vi "control_excitadores.vi"(4 "Action":u32, 5 "AL TX 1":bool caption="AL TX", 7 "COM DATA":T1={"IP "="192.168.1.7", "Puerto:"=2101, "Time Out"=800}) -> (1 "error out":errorcluster)   [LabVIEW 2010]
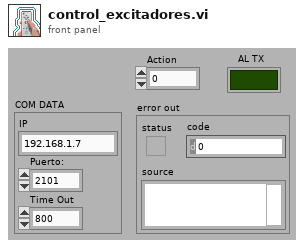
[diagram p1: front panel]
types:
  T1 = cluster{"IP ":string, "Puerto:":u16, "Time Out":u16}
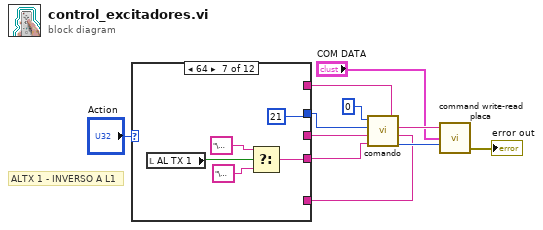
[diagram p0: block diagram]
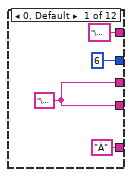
[diagram p2: hidden frame]
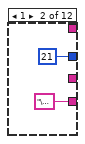
[diagram p3: hidden frame]
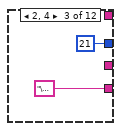
[diagram p4: hidden frame]
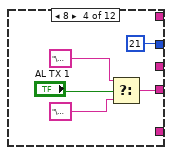
[diagram p5: hidden frame]
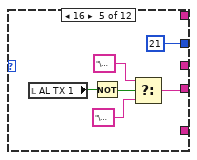
[diagram p6: hidden frame]
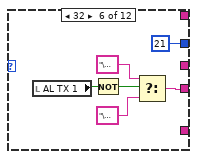
[diagram p7: hidden frame]
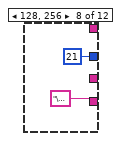
[diagram p8: hidden frame]
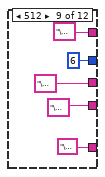
[diagram p9: hidden frame]
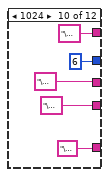
[diagram p10: hidden frame]
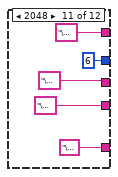
[diagram p11: hidden frame]
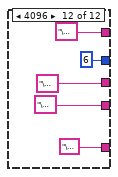
[diagram p12: hidden frame]
diagram:
  # "ALTX 1 - INVERSO A L1"
  n1 = case shown="64" "Action" {
    tunnel: [w15 _ _ _ _ _ _ _ "\u0003" ("ANEXO H") "\u0003" ("ANEXO H") "\u0003" ("ANEXO H") "\u0003" ("ANEXO H")] -> w6
    tunnel: [w15 "\u0006" ("LOW") "\u0007" ("LOW") w20 w26 w31 w37 "\u0001" ("LOW") "\u0000" ("ANEXO H") "\u0000" ("ANEXO H") "\u0000" ("ANEXO H") "\u0000" ("ANEXO H")] -> w5
    tunnel: ["\u0004" ("ANEXO H") _ _ _ _ _ _ _ "\u0000" ("ANEXO H") "\u0001" ("ANEXO H") "\u0002" ("ANEXO H") "\u0003" ("ANEXO H")] -> w4
    tunnel: ["À" ("LOW") _ _ _ _ _ _ _ "\u0000" ("LOW") "\u0000" ("LOW") "\u0000" ("LOW") "\u0000" ("LOW")] -> w3
    tunnel: [u8 6 ("Comando:") u8 21 ("Comando:") u8 21 ("Comando:") u8 21 ("Comando:") u8 21 ("Comando:") u8 21 ("Comando:") u8 21 ("Comando:") u8 21 ("Comando:") u8 6 ("Comando:") u8 6 ("Comando:") u8 6 ("Comando:") u8 6 ("Comando:")] -> w1
    frame 0, Default {
      w15 = "\u0000" ("LOW")
    }
    frame 1 {
    }
    frame 2, 4 {
    }
    frame 8 {
      n2 = Select(t="\u0005" ("ANEXO H"), s="AL TX 1", f="\u0004" ("ANEXO H")) -> (s? t:f=w20:string)
    }
    frame 16 {
      n3 = local read "AL TX 1"() -> (w27:bool)
      n4 = Not(x=w27) -> (.not. x?=w28:bool)
      n5 = Select(t="\u0002" ("ANEXO H"), s=w28, f="\u0003" ("ANEXO H")) -> (s? t:f=w26:string)
    }
    frame 32 {
      n6 = local read "AL TX 1"() -> (w34:bool)
      n7 = Not(x=w34) -> (.not. x?=w33:bool)
      n8 = Select(t="\u0005" ("ANEXO H"), s=w33, f="\u0004" ("ANEXO H")) -> (s? t:f=w31:string)
    }
    frame 64 {
      n9 = local read "AL TX 1"() -> (w41:bool)
      n10 = Select(t="\u0002" ("ANEXO H"), s=w41, f="\u0003" ("ANEXO H")) -> (s? t:f=w37:string)
    }
    frame 128, 256 {
    }
    frame 512 {
    }
    frame 1024 {
    }
    frame 2048 {
    }
    frame 4096 {
    }
  }
  n11 = call "comando.vi"("ANEXO L"=w3, "ANEXO H"=w4, "LOW"=w5, "HIGH"=w6, "Comando:"=w1, "Equipo Nº"=u8 0 ("Comando:")) -> ("Bytes OUT"=w9:u16, "comando"=w8:string)  [unwired: 1 in]
  n12 = call "command write-read placa.vi"("Write Command"=w8, "COM DATA"="COM DATA", "bytes"=w9) -> ("error out"=→"error out":errorcluster)  [unwired: 3 in, 1 out]
